vi "youtubeDemoDropDownMenu.vi"() -> ()   [LabVIEW 2020]
panel:
  in  "Ring":u16(ring) items=["Turn off the light", "Turn on the light", "SOS", "hip hop", "Movie lighting", "sunlight", "moonlight", "starlight"]
  in  "Enum":T1(ring)
  in  "Stop the program":bool
  out "My Text":string
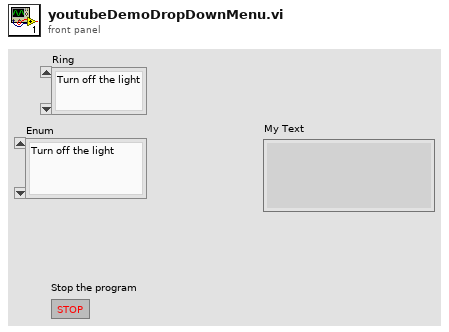
[diagram p1: front panel]
types:
  T1 = enum16{"Turn off the light", "Turn on the light", "SOS", "hip hop", "Movie lighting", "sunlight", "moonlight", "starlight"}
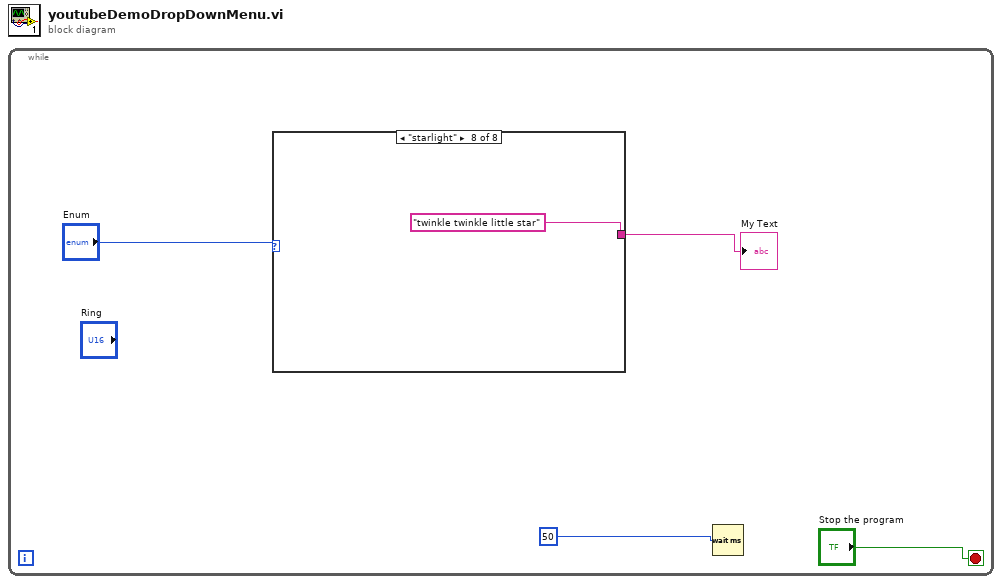
[diagram p0: block diagram]
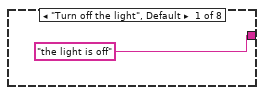
[diagram p2: hidden frame]
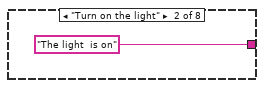
[diagram p3: hidden frame]
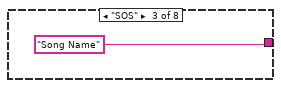
[diagram p4: hidden frame]
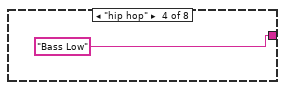
[diagram p5: hidden frame]
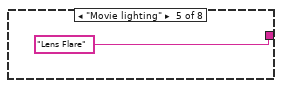
[diagram p6: hidden frame]
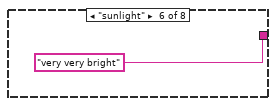
[diagram p7: hidden frame]
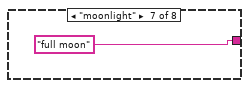
[diagram p8: hidden frame]
diagram:
  n1 = while {
    stop <- "Stop the program" stop-if-true
    n2 = case shown="\"starlight\"" "Enum" {
      tunnel: ["the light is off" "The light  is on" "Song Name" "Bass Low" "Lens Flare" "very very bright" "full moon" "twinkle twinkle little star"] -> w4
      frame "Turn off the light", Default {
      }
      frame "Turn on the light" {
      }
      frame "SOS" {
      }
      frame "hip hop" {
      }
      frame "Movie lighting" {
      }
      frame "sunlight" {
      }
      frame "moonlight" {
      }
      frame "starlight" {
      }
    }
    "My Text" <- w4
    n3 = Wait (ms)(milliseconds to wait=50) -> ()  [unwired: 1 out]
  }
